vi "Exit DataBase.vi"(8 "error in (no error)":errorcluster, 11 "connection reference":T1) -> (0 "error out":errorcluster)   [LabVIEW 2014]
uses:
  <vilib>/addons/database/NI_Database_API.lvlib
  <vilib>/addons/database/Connection.llb/Conn ObjectReference.ctl
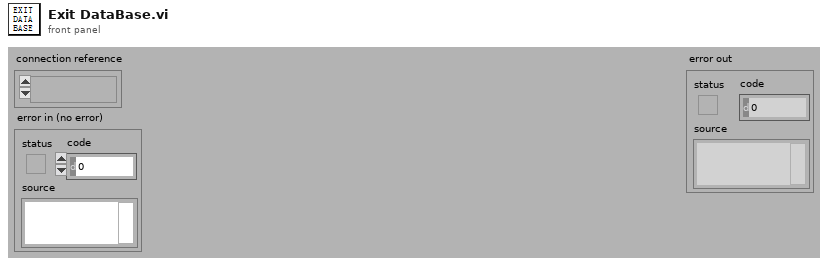
[diagram p1: front panel]
types:
  T1 = typedef "NI_Database_API.lvlib/Conn ObjectReference.ctl" = refnum<k1>
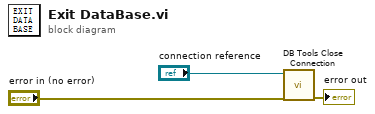
[diagram p0: block diagram]
diagram:
  n1 = call <vilib>:"DB Tools Close Connection.vi"("error in (no error)"="error in (no error)", "connection reference"="connection reference") -> ("error out"=→"error out":errorcluster)  [unwired: 5 in]
